vi "CAN STP Engine Reference Create.vi"(8 "error in":errorcluster, 11 "Selected Sockets":i16[](array[numeric])) -> (0 "error out":errorcluster)   [LabVIEW 2023, in "LTT_TeststandSteptypes.lvlib"]
uses:
  LTT_TeststandSteptypes.lvlib
  Control/CAN FGV State.ctl
  STP Engine SubVI/Control/STP Engine Rx Data.ctl
  HardwareAbstractionLayer_LVOOP/CAN/CAN Application Protocols/STP Protocol_class/Ctrls/STP Output Data.ctl
  HardwareAbstractionLayer_LVOOP/CAN/CAN Application Protocols/STP Protocol_class/Ctrls/STP Error Cluster.ctl
  STP Engine SubVI/Control/STP Engine Tx Data.ctl
  HardwareAbstractionLayer_LVOOP/CAN/CAN Application Protocols/STP Protocol_class/Ctrls/STP Input Data.ctl
  HardwareAbstractionLayer_LVOOP/CAN/CAN Application Protocols/STP Protocol_class/Ctrls/STP CMD.ctl
  HardwareAbstractionLayer_LVOOP/CAN/CAN Application Protocols/STP Protocol_class/STP Protocol.lvclass
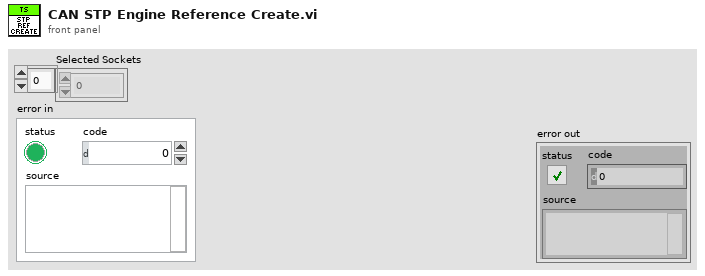
[diagram p1: front panel]
types:
  T1 = typedef "LTT_TeststandSteptypes.lvlib/CAN FGV State.ctl" = enum16{"Init", "Get", "Set"}
  T2 = typedef "LTT_TeststandSteptypes.lvlib/STP Engine Tx Data.ctl" = cluster{"STP Input Data":T3, "Socket No":u16}
  T3 = typedef "HardwareAbstractionLayer_LVOOP.lvlib/CAN Application Protocols Lib.lvlib/STP Protocol.lvclass/STP Input Data.ctl" = cluster{"TxID":u32, "RxID":u32, "CMD":T4, "RQ Data":u8[], "+veResponseCode":u8, "ResponseTimeout (S)":dbl}
  T4 = typedef "HardwareAbstractionLayer_LVOOP.lvlib/CAN Application Protocols Lib.lvlib/STP Protocol.lvclass/STP CMD.ctl" = u8
  T5 = typedef "LTT_TeststandSteptypes.lvlib/STP Engine Rx Data.ctl" = cluster{"STP Output Data":T6, "RequestTimeout?":bool}
  T6 = typedef "HardwareAbstractionLayer_LVOOP.lvlib/CAN Application Protocols Lib.lvlib/STP Protocol.lvclass/STP Output Data.ctl" = cluster{"ResponseData":u8[], "ResponseData(ASCII)":string, "PositiveResponse?":bool, "STP Error":T7}
  T7 = typedef "HardwareAbstractionLayer_LVOOP.lvlib/CAN Application Protocols Lib.lvlib/STP Protocol.lvclass/STP Error Cluster.ctl" = cluster{"Status":bool, "Code":u8, "Error":string, "Description":string}
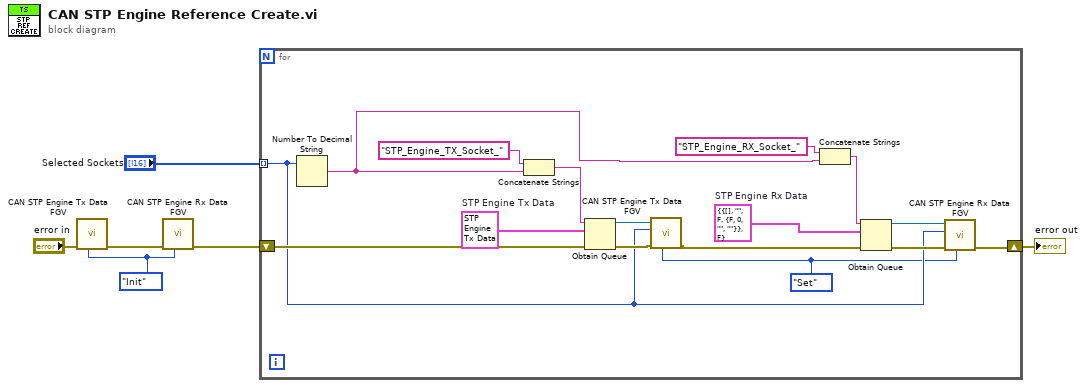
[diagram p0: block diagram]
diagram:
  w4 = CAN_FGV_State."Init" ("CAN FGV State")
  n1 = call "CAN STP Engine Tx Data FGV.vi"("CAN FGV State"=w4, "error in"="error in") -> ("error out"=w6:errorcluster)  [unwired: 7 in, 2 out]
  n2 = call "CAN STP Engine Rx Data FGV.vi"("CAN FGV State"=w4, "error in"=w6) -> ("error out"=w5:errorcluster)  [unwired: 8 in, 1 out]
  n3 = for {
    tunnel: "Selected Sockets" -> [w10] mode=indexing
    shift-right: [w8] -> w2
    shift-left: w5 -> [w16]
    w9 = CAN_FGV_State."Set" ("CAN FGV State")
    w21 = T2 {"STP Input Data"={"TxID"=2042, "RxID"=2043, "CMD"=130, "RQ Data"=[], "+veResponseCode"=160, "ResponseTimeout (S)"=1.0}, "Socket No"=0}  # STP Engine Tx Data
    w19 = T5 {"STP Output Data"={"ResponseData"=[], "ResponseData(ASCII)"="", "PositiveResponse?"=FALSE, "STP Error"={"Status"=FALSE, "Code"=0, "Error"="", "Description"=""}}, "RequestTimeout?"=FALSE}  # STP Engine Rx Data
    n4 = Number To Decimal String(number=w10) -> (decimal integer string=w15:string)  [unwired: 1 in]
    n5 = Concatenate Strings("STP_Engine_TX_Socket_", w15) -> (w20:string)
    n6 = Obtain Queue(name (unnamed)=w20, element data type=w21, error in (no error)=w16) -> (queue out=w7:refnum<queue>, error out=w14:errorcluster)  [unwired: 2 in, 1 out]
    n7 = call "CAN STP Engine Tx Data FGV.vi"("CAN FGV State"=w9, "error in"=w14, "Socket No"=w10, "STP Engine Tx Data in"=w7) -> ("error out"=w13:errorcluster)  [unwired: 5 in, 2 out]
    n8 = Concatenate Strings("STP_Engine_RX_Socket_", w15) -> (w17:string)
    n9 = Obtain Queue(name (unnamed)=w17, element data type=w19, error in (no error)=w13) -> (queue out=w11:refnum<queue>, error out=w12:errorcluster)  [unwired: 2 in, 1 out]
    n10 = call "CAN STP Engine Rx Data FGV.vi"("CAN FGV State"=w9, "error in"=w12, "Socket No"=w10, "STP Engine Rx Data in"=w11) -> ("error out"=w8:errorcluster)  [unwired: 6 in, 1 out]
  }
  "error out" <- w2
